vi "TankSystem.vi"(0 "Input":dbl) -> (1 "Output":bool, 2 "Tank":dbl(slide) scale=0.0..50.0)   [LabVIEW 2020]
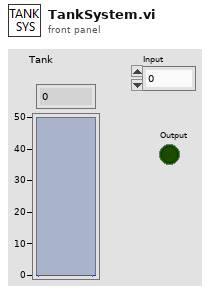
[diagram p1: front panel]
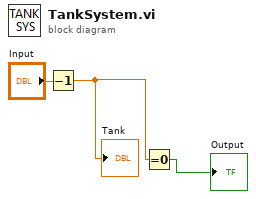
[diagram p0: block diagram]
diagram:
  n1 = Decrement(x="Input") -> (x-1=w3:dbl)
  "Tank" <- w3
  n2 = Equal To 0?(x=w3) -> (x = 0?=→"Output":bool)
